vi "Configure Pulse Waveform.vi"(8 "error in (no error)":errorcluster, 9 "Duty Cycle (50%)":dbl=50.0, 10 "Channel (1: Channel 1)":u16(ring)=1 items=["Channel 1"=1, "Channel 2"=2], 11 "VISA resource name":refnum<visa-resource-name>) -> (0 "error out":errorcluster, 3 "VISA resource name out":refnum<visa-resource-name>)   [LabVIEW 2016, in "Tektronix AFG 1000 Series.lvlib"]
doc: "Configures the duty cycle of the pulse waveform for the specified channel."
uses:
  Tektronix AFG 1000 Series.lvlib
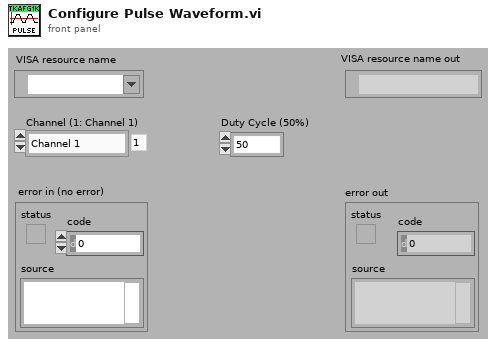
[diagram p1: front panel]
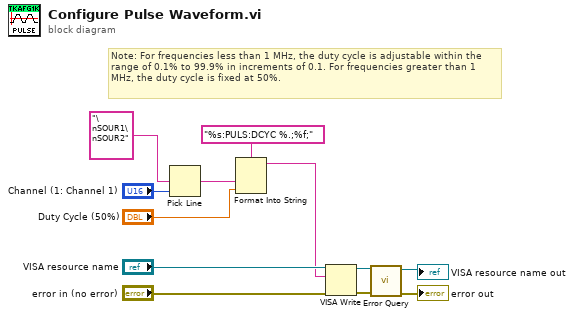
[diagram p0: block diagram]
diagram:
  # "Note: For frequencies less than 1 MHz, the duty cycle is adjustable within the range of 0.1% to 99.9% in increments of 0.1. For frequencies greater than 1 MHz, the duty cycle is fixed at 50%."
  n1 = Pick Line(multi-line string="\nSOUR1\nSOUR2" ("string (\"\")"), line index="Channel (1: Channel 1)") -> (output string=w2:string)  [unwired: 1 in]
  n2 = Format Into String(format string="%s:PULS:DCYC %.;%f;", w2, "Duty Cycle (50%)") -> (resulting string=w1:string)  [unwired: 2 in, 1 out]
  n3 = VISA Write(VISA resource name="VISA resource name", write buffer=w1, error in (no error)="error in (no error)") -> (VISA resource name out=w10:refnum<visa-resource-name>, error out=w9:errorcluster)  [unwired: 1 out]
  n4 = call "Error Query.vi"("error in (no error)"=w9, "VISA resource name"=w10) -> ("error out"=→"error out":errorcluster, "VISA resource name out"=→"VISA resource name out":refnum<visa-resource-name>)  [unwired: 6 in, 2 out]
